vi "ReadData.vi"(8 "error in":errorcluster, 11 "Module Config Selector":i16) -> (0 "error out":errorcluster, 1 "Number Of Pulses":u32, 2 "OversampleClk Ticks":u32, 3 "Data Array":sgl[](array[numeric]) format="%.2f")   [LabVIEW 2017, in "VDMS_VibAPI.lvlib"]
uses:
  <vilib>/addons/InsightCM/Devices/Shared/Cms/Fpga/AcquisitionFpgaTach/source/subVIs/VibAPI/VDMS_VibAPI.lvlib
  <vilib>/rvi/eio/common/nirviEmuTemplateMethod_errors.vi
  <vilib>/rvi/Memory/Memory_Emulation/nirvimemoryFastEmulation.vi
  <vilib>/rvi/Memory/Memory_Emulation/nirvimemoryEmulation.vi
  <vilib>/rvi/Emulation/niFpgaEmulationIsFPGAContextNoSignature.vi
  <vilib>/rvi/DataTransferAndStorage/Container/Common/niFpgaContainerGetUniqueNameForEmu.vi
  <vilib>/rvi/Emulation/niFpgaProcessEmulError.vi
  <vilib>/rvi/Emulation/niFpgaSctlEmulationGetInTimedLoop.vi
  <vilib>/rvi/errors/nirviReportUnexpectedCaseInternalError (U32).vi
  <vilib>/eio/EIONode/EIONode.xnode
  <vilib>/rvi/DataTransferAndStorage/Container/XNode/niFpgaContainer.xnode
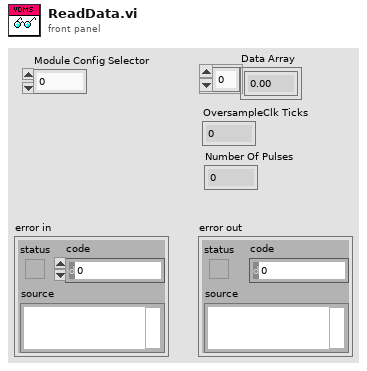
[diagram p1: front panel]
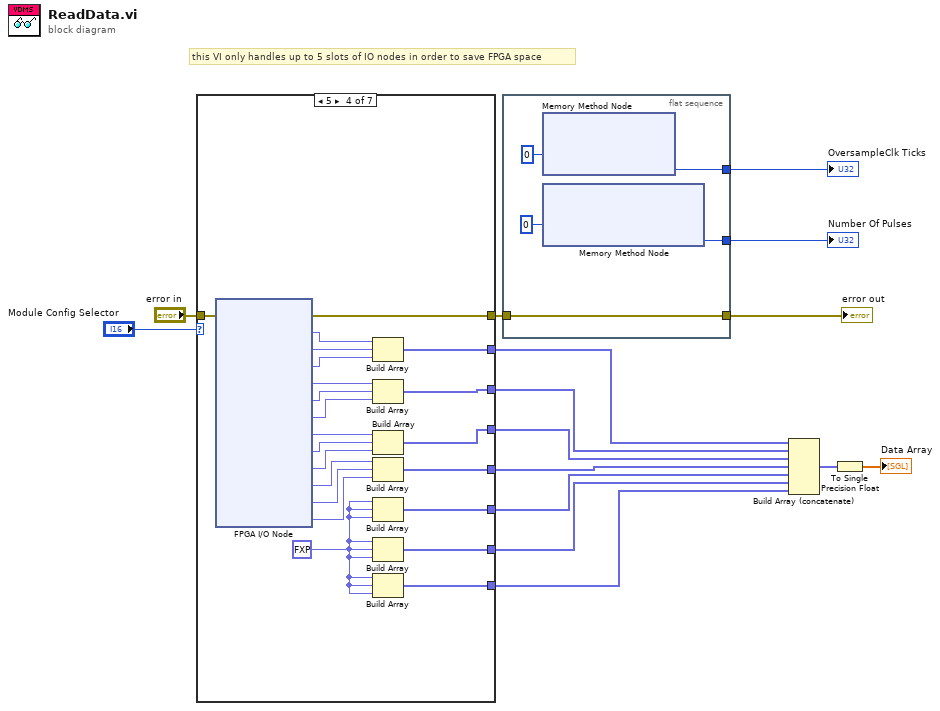
[diagram p0: block diagram]
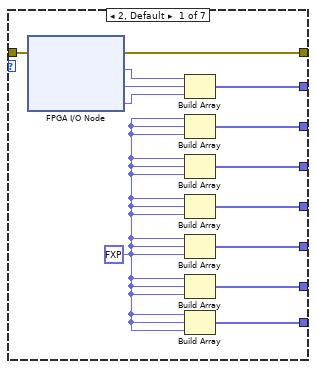
[diagram p2: hidden frame]
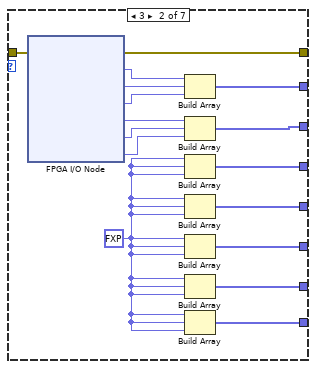
[diagram p3: hidden frame]
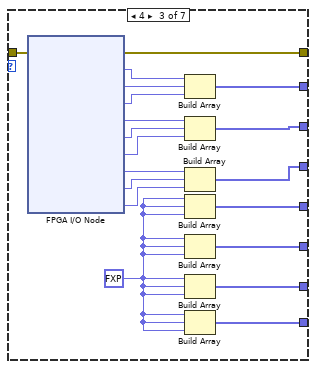
[diagram p4: hidden frame]
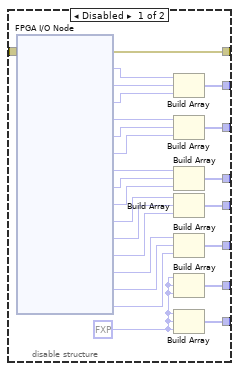
[diagram p6: hidden frame]
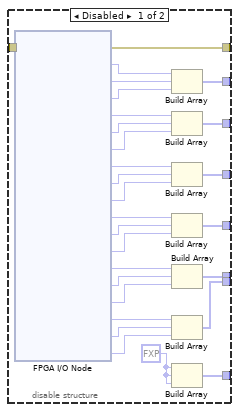
[diagram p8: hidden frame]
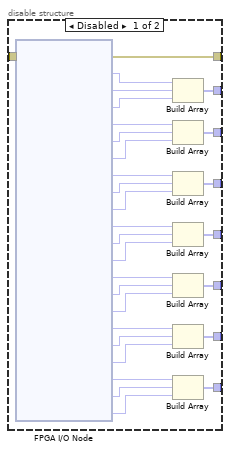
[diagram p10: hidden frame]
diagram:
  # "this VI only handles up to 5 slots of IO nodes in order to save FPGA space"
  n1 = case shown="5" "Module Config Selector" {
    tunnel: "error in" -> [w28 w44 w63 w85 w94 w129 w167]
    tunnel: [w27 w43 w62 w84 w93 w128 w166] -> w6
    tunnel: [w26 w42 w61 w83 w92 w127 w165] -> w14
    tunnel: [w25 w41 w60 w82 w91 w126 w164] -> w13
    tunnel: [w24 w40 w59 w81 w90 w125 w163] -> w12
    tunnel: [w23 w39 w58 w80 w89 w124 w162] -> w11
    tunnel: [w22 w38 w57 w79 w88 w123 w161] -> w10
    tunnel: [w18 w31 w47 w78 w87 w122 w160] -> w8
    tunnel: [w16 w29 w45 w77 w86 w121 w159] -> w7
    frame 2, Default {
      w17 = fxp<+/-,24,7> 0.0 ("Mod1/AI2")
      n2 = xnode "FPGA I/O Node"("error in"=w28) -> ("error out"=w27:errorcluster, "Mod2/AI0"=w21:fxp<+/-,24,7>, "Mod2/AI1"=w20:fxp<+/-,24,7>, "Mod2/AI2"=w19:fxp<+/-,24,7>)  [unwired: 3 in, 3 out]
      n3 = Build Array(w21, w20, w19) -> (w26:fxp<+/-,24,7>[])
      n4 = Build Array(w17, w17, w17) -> (w25:fxp<+/-,24,7>[])
      n5 = Build Array(w17, w17, w17) -> (w24:fxp<+/-,24,7>[])
      n6 = Build Array(w17, w17, w17) -> (w23:fxp<+/-,24,7>[])
      n7 = Build Array(w17, w17, w17) -> (w22:fxp<+/-,24,7>[])
      n8 = Build Array(w17, w17, w17) -> (w18:fxp<+/-,24,7>[])
      n9 = Build Array(w17, w17, w17) -> (w16:fxp<+/-,24,7>[])
    }
    frame 3 {
      w30 = fxp<+/-,24,7> 0.0 ("Mod1/AI2")
      n10 = xnode "FPGA I/O Node"("error in"=w44) -> ("error out"=w43:errorcluster, "Mod2/AI0"=w37:fxp<+/-,24,7>, "Mod2/AI1"=w36:fxp<+/-,24,7>, "Mod2/AI2"=w35:fxp<+/-,24,7>, "Mod3/AI0"=w34:fxp<+/-,24,7>, "Mod3/AI1"=w33:fxp<+/-,24,7>, "Mod3/AI2"=w32:fxp<+/-,24,7>)  [unwired: 6 in, 6 out]
      n11 = Build Array(w37, w36, w35) -> (w42:fxp<+/-,24,7>[])
      n12 = Build Array(w34, w33, w32) -> (w41:fxp<+/-,24,7>[])
      n13 = Build Array(w30, w30, w30) -> (w40:fxp<+/-,24,7>[])
      n14 = Build Array(w30, w30, w30) -> (w39:fxp<+/-,24,7>[])
      n15 = Build Array(w30, w30, w30) -> (w38:fxp<+/-,24,7>[])
      n16 = Build Array(w30, w30, w30) -> (w31:fxp<+/-,24,7>[])
      n17 = Build Array(w30, w30, w30) -> (w29:fxp<+/-,24,7>[])
    }
    frame 4 {
      w46 = fxp<+/-,24,7> 0.0 ("Mod1/AI2")
      n18 = xnode "FPGA I/O Node"("error in"=w63) -> ("error out"=w62:errorcluster, "Mod2/AI0"=w56:fxp<+/-,24,7>, "Mod2/AI1"=w55:fxp<+/-,24,7>, "Mod2/AI2"=w54:fxp<+/-,24,7>, "Mod3/AI0"=w53:fxp<+/-,24,7>, "Mod3/AI1"=w52:fxp<+/-,24,7>, "Mod3/AI2"=w51:fxp<+/-,24,7>, "Mod4/AI0"=w50:fxp<+/-,24,7>, "Mod4/AI1"=w49:fxp<+/-,24,7>, "Mod4/AI2"=w48:fxp<+/-,24,7>)  [unwired: 9 in, 9 out]
      n19 = Build Array(w56, w55, w54) -> (w61:fxp<+/-,24,7>[])
      n20 = Build Array(w53, w52, w51) -> (w60:fxp<+/-,24,7>[])
      n21 = Build Array(w50, w49, w48) -> (w59:fxp<+/-,24,7>[])
      n22 = Build Array(w46, w46, w46) -> (w58:fxp<+/-,24,7>[])
      n23 = Build Array(w46, w46, w46) -> (w57:fxp<+/-,24,7>[])
      n24 = Build Array(w46, w46, w46) -> (w47:fxp<+/-,24,7>[])
      n25 = Build Array(w46, w46, w46) -> (w45:fxp<+/-,24,7>[])
    }
    frame 5 {
      w64 = fxp<+/-,24,7> 0.0 ("Mod1/AI2")
      n26 = xnode "FPGA I/O Node"("error in"=w85) -> ("error out"=w84:errorcluster, "Mod2/AI0"=w76:fxp<+/-,24,7>, "Mod2/AI1"=w75:fxp<+/-,24,7>, "Mod2/AI2"=w74:fxp<+/-,24,7>, "Mod3/AI0"=w73:fxp<+/-,24,7>, "Mod3/AI1"=w72:fxp<+/-,24,7>, "Mod3/AI2"=w71:fxp<+/-,24,7>, "Mod4/AI0"=w70:fxp<+/-,24,7>, "Mod4/AI1"=w69:fxp<+/-,24,7>, "Mod4/AI2"=w68:fxp<+/-,24,7>, "Mod5/AI0"=w67:fxp<+/-,24,7>, "Mod5/AI1"=w66:fxp<+/-,24,7>, "Mod5/AI2"=w65:fxp<+/-,24,7>)  [unwired: 12 in, 12 out]
      n27 = Build Array(w76, w75, w74) -> (w83:fxp<+/-,24,7>[])
      n28 = Build Array(w73, w72, w71) -> (w82:fxp<+/-,24,7>[])
      n29 = Build Array(w70, w69, w68) -> (w81:fxp<+/-,24,7>[])
      n30 = Build Array(w67, w66, w65) -> (w80:fxp<+/-,24,7>[])
      n31 = Build Array(w64, w64, w64) -> (w79:fxp<+/-,24,7>[])
      n32 = Build Array(w64, w64, w64) -> (w78:fxp<+/-,24,7>[])
      n33 = Build Array(w64, w64, w64) -> (w77:fxp<+/-,24,7>[])
    }
    frame 6 {
      n34 = disable-structure shown="Enabled" {
        disable-tunnel: w94 -> [w119 w120]
        disable-tunnel: [w118 w120] -> w93
        disable-tunnel: [w117 _] -> w92
        disable-tunnel: [w116 _] -> w91
        disable-tunnel: [w115 _] -> w90
        disable-tunnel: [w114 _] -> w89
        disable-tunnel: [w113 _] -> w88
        disable-tunnel: [w97 _] -> w87
        disable-tunnel: [w95 _] -> w86
        frame Disabled {
          w96 = fxp<+/-,24,7> 0.0 ("Mod1/AI2")
          n35 = xnode "FPGA I/O Node"("error in"=w119) -> ("error out"=w118:errorcluster, "Mod2/AI0"=w112:fxp<+/-,24,7>, "Mod2/AI1"=w111:fxp<+/-,24,7>, "Mod2/AI2"=w110:fxp<+/-,24,7>, "Mod3/AI0"=w109:fxp<+/-,24,7>, "Mod3/AI1"=w108:fxp<+/-,24,7>, "Mod3/AI2"=w107:fxp<+/-,24,7>, "Mod4/AI0"=w106:fxp<+/-,24,7>, "Mod4/AI1"=w105:fxp<+/-,24,7>, "Mod4/AI2"=w104:fxp<+/-,24,7>, "Mod5/AI0"=w103:fxp<+/-,24,7>, "Mod5/AI1"=w102:fxp<+/-,24,7>, "Mod5/AI2"=w101:fxp<+/-,24,7>, "Mod6/AI0"=w100:fxp<+/-,24,7>, "Mod6/AI1"=w99:fxp<+/-,24,7>, "Mod6/AI2"=w98:fxp<+/-,24,7>)  [unwired: 15 in, 15 out]
          n36 = Build Array(w112, w111, w110) -> (w117:fxp<+/-,24,7>[])
          n37 = Build Array(w109, w108, w107) -> (w116:fxp<+/-,24,7>[])
          n38 = Build Array(w106, w105, w104) -> (w115:fxp<+/-,24,7>[])
          n39 = Build Array(w103, w102, w101) -> (w114:fxp<+/-,24,7>[])
          n40 = Build Array(w100, w99, w98) -> (w113:fxp<+/-,24,7>[])
          n41 = Build Array(w96, w96, w96) -> (w97:fxp<+/-,24,7>[])
          n42 = Build Array(w96, w96, w96) -> (w95:fxp<+/-,24,7>[])
        }
        frame Enabled {
        }
      }
    }
    frame 7 {
      n43 = disable-structure shown="Enabled" {
        disable-tunnel: w129 -> [w157 w158]
        disable-tunnel: [w156 w158] -> w128
        disable-tunnel: [w155 _] -> w127
        disable-tunnel: [w154 _] -> w126
        disable-tunnel: [w153 _] -> w125
        disable-tunnel: [w152 _] -> w124
        disable-tunnel: [w151 _] -> w123
        disable-tunnel: [w150 _] -> w122
        disable-tunnel: [w149 _] -> w121
        frame Disabled {
          w130 = fxp<+/-,24,7> 0.0 ("Mod1/AI2")
          n44 = xnode "FPGA I/O Node"("error in"=w157) -> ("error out"=w156:errorcluster, "Mod2/AI0"=w134:fxp<+/-,24,7>, "Mod2/AI1"=w135:fxp<+/-,24,7>, "Mod2/AI2"=w136:fxp<+/-,24,7>, "Mod3/AI0"=w137:fxp<+/-,24,7>, "Mod3/AI1"=w138:fxp<+/-,24,7>, "Mod3/AI2"=w139:fxp<+/-,24,7>, "Mod4/AI0"=w140:fxp<+/-,24,7>, "Mod4/AI1"=w141:fxp<+/-,24,7>, "Mod4/AI2"=w142:fxp<+/-,24,7>, "Mod5/AI0"=w143:fxp<+/-,24,7>, "Mod5/AI1"=w144:fxp<+/-,24,7>, "Mod5/AI2"=w145:fxp<+/-,24,7>, "Mod6/AI0"=w146:fxp<+/-,24,7>, "Mod6/AI1"=w147:fxp<+/-,24,7>, "Mod6/AI2"=w148:fxp<+/-,24,7>, "Mod7/AI0"=w133:fxp<+/-,24,7>, "Mod7/AI1"=w132:fxp<+/-,24,7>, "Mod7/AI2"=w131:fxp<+/-,24,7>)  [unwired: 18 in, 18 out]
          n45 = Build Array(w134, w135, w136) -> (w155:fxp<+/-,24,7>[])
          n46 = Build Array(w137, w138, w139) -> (w154:fxp<+/-,24,7>[])
          n47 = Build Array(w140, w141, w142) -> (w153:fxp<+/-,24,7>[])
          n48 = Build Array(w143, w144, w145) -> (w152:fxp<+/-,24,7>[])
          n49 = Build Array(w146, w147, w148) -> (w151:fxp<+/-,24,7>[])
          n50 = Build Array(w133, w132, w131) -> (w150:fxp<+/-,24,7>[])
          n51 = Build Array(w130, w130, w130) -> (w149:fxp<+/-,24,7>[])
        }
        frame Enabled {
        }
      }
    }
    frame 8 {
      n52 = disable-structure shown="Enabled" {
        disable-tunnel: w167 -> [w197 w198]
        disable-tunnel: [w196 w198] -> w166
        disable-tunnel: [w195 _] -> w165
        disable-tunnel: [w194 _] -> w164
        disable-tunnel: [w193 _] -> w163
        disable-tunnel: [w192 _] -> w162
        disable-tunnel: [w191 _] -> w161
        disable-tunnel: [w190 _] -> w160
        disable-tunnel: [w189 _] -> w159
        frame Disabled {
          n53 = xnode "FPGA I/O Node"("error in"=w197) -> ("error out"=w196:errorcluster, "Mod2/AI0"=w174:fxp<+/-,24,7>, "Mod2/AI1"=w175:fxp<+/-,24,7>, "Mod2/AI2"=w176:fxp<+/-,24,7>, "Mod3/AI0"=w177:fxp<+/-,24,7>, "Mod3/AI1"=w178:fxp<+/-,24,7>, "Mod3/AI2"=w179:fxp<+/-,24,7>, "Mod4/AI0"=w180:fxp<+/-,24,7>, "Mod4/AI1"=w181:fxp<+/-,24,7>, "Mod4/AI2"=w182:fxp<+/-,24,7>, "Mod5/AI0"=w183:fxp<+/-,24,7>, "Mod5/AI1"=w184:fxp<+/-,24,7>, "Mod5/AI2"=w185:fxp<+/-,24,7>, "Mod6/AI0"=w186:fxp<+/-,24,7>, "Mod6/AI1"=w187:fxp<+/-,24,7>, "Mod6/AI2"=w188:fxp<+/-,24,7>, "Mod7/AI0"=w173:fxp<+/-,24,7>, "Mod7/AI1"=w172:fxp<+/-,24,7>, "Mod7/AI2"=w171:fxp<+/-,24,7>, "Mod8/AI0"=w170:fxp<+/-,24,7>, "Mod8/AI1"=w169:fxp<+/-,24,7>, "Mod8/AI2"=w168:fxp<+/-,24,7>)  [unwired: 21 in, 21 out]
          n54 = Build Array(w174, w175, w176) -> (w195:fxp<+/-,24,7>[])
          n55 = Build Array(w177, w178, w179) -> (w194:fxp<+/-,24,7>[])
          n56 = Build Array(w180, w181, w182) -> (w193:fxp<+/-,24,7>[])
          n57 = Build Array(w183, w184, w185) -> (w192:fxp<+/-,24,7>[])
          n58 = Build Array(w186, w187, w188) -> (w191:fxp<+/-,24,7>[])
          n59 = Build Array(w173, w172, w171) -> (w190:fxp<+/-,24,7>[])
          n60 = Build Array(w170, w169, w168) -> (w189:fxp<+/-,24,7>[])
        }
        frame Enabled {
        }
      }
    }
  }
  n61 = flat-sequence {
    tunnel: w6 -> [w203]
    tunnel: [w203] -> w5
    tunnel: [w202] -> w2
    tunnel: [w199] -> w1
    frame #0 {
      n62 = xnode ("Memory Method Node")("Address"=u32 0) -> ("Data"=w202:u32)  [unwired: 1 in, 1 out]
      n63 = xnode ("Memory Method Node")("Address"=u32 0) -> ("Data"=w199:u32)  [unwired: 1 in, 1 out]
    }
  }
  n64 = Build Array (concatenate)(w14, w13, w12, w11, w10, w8, w7) -> (w4:fxp<+/-,24,7>[])
  n65 = To Single Precision Float(number=w4) -> (single precision float=→"Data Array":sgl[])
  "error out" <- w5
  "OversampleClk Ticks" <- w2
  "Number Of Pulses" <- w1
